vi "Forward_conVAE.vi"(6 "X":sgl[][](array[numeric]), 7 "Y":sgl[][](array[numeric]), 8 "validate":bool=TRUE, 9 "ptr_decoder":i64, 10 "ptr_encoder":i64, 11 "error in (no error)":errorcluster) -> (1 "X_HAT":sgl[][](array[numeric]), 2 "error":sgl, 3 "error out":errorcluster)   [LabVIEW 2016, in "CNet.lvlib"]
uses:
  CNet.lvlib
  Users/jg754/Documents/Visual Studio 2015/Projects/CLearn/x64/Release/CLearn.dll
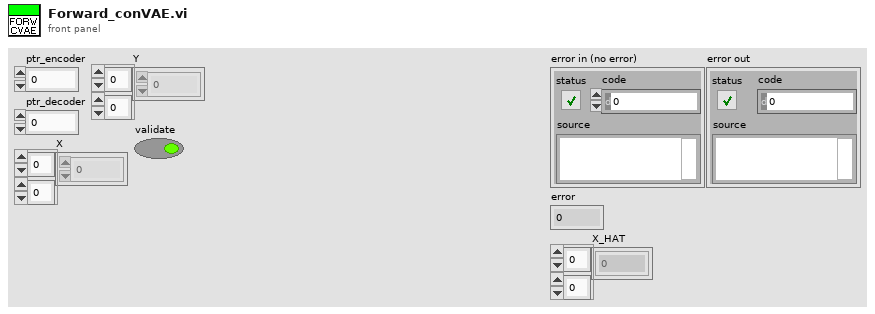
[diagram p1: front panel]
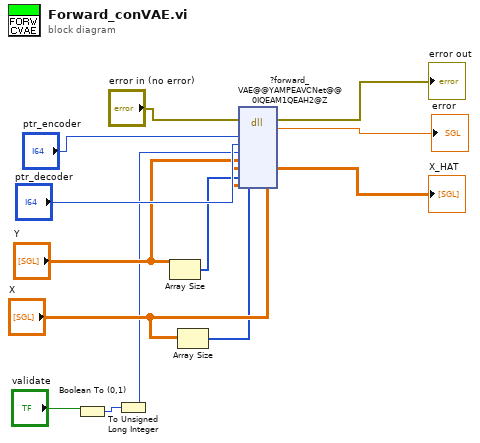
[diagram p0: block diagram]
diagram:
  n1 = Boolean To (0,1)(Boolean="validate") -> (0, 1=w2:i16)
  n2 = To Unsigned Long Integer(number=w2) -> (unsigned 32bit integer=w1:u32)
  n3 = Array Size(array="Y") -> (size(s)=w7:i32[])
  n4 = Array Size(array="X") -> (size(s)=w5:i32[])
  n5 = dll-call lib="C:/Users/jg754/Documents/Visual Studio 2015/Projects/CLearn/x64/Release/CLearn.dll" fn="?forward_VAE@@YAMPEAVCNet@@0IQEAM1QEAH2@Z"(error in="error in (no error)", "ptr_encoder"="ptr_encoder", "ptr_decoder"="ptr_decoder", "validate"=w1, "Y"="Y", "X"="X", "Y_format"=w7, "X_format"=w5) -> (error out=→"error out":errorcluster, "error"=→"error":sgl, "X"=→"X_HAT":sgl[][])  [unwired: 8 in, 1 out]
